vi "Normalize.vi"(8 "error in":errorcluster, 11 "Source graph":cluster{dbl[], dbl[]}[](graph)) -> (0 "error out":errorcluster, 3 "Normalized source graph out":cluster{dbl[], dbl[]}[](graph))   [LabVIEW 2024]
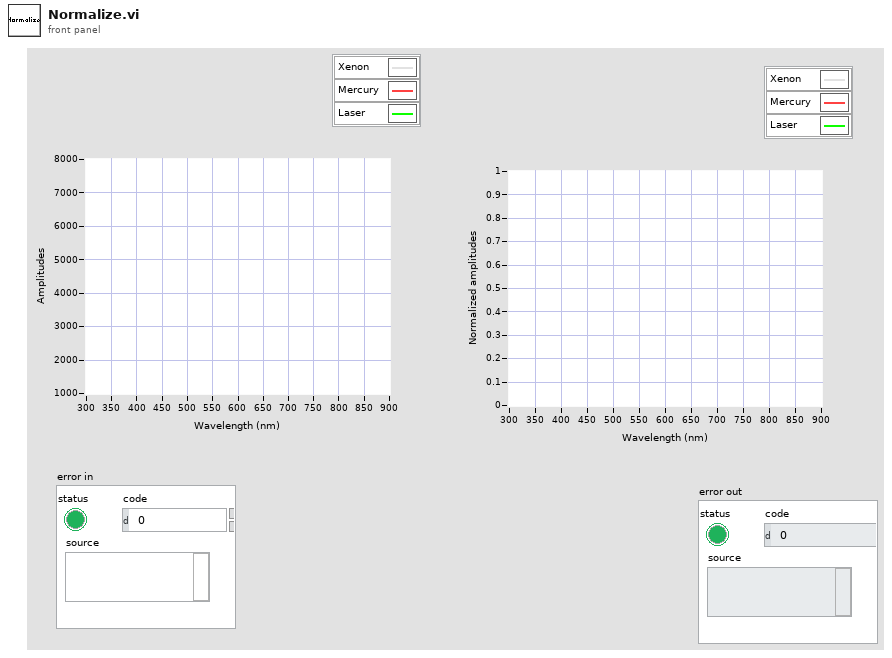
[diagram p1: front panel]
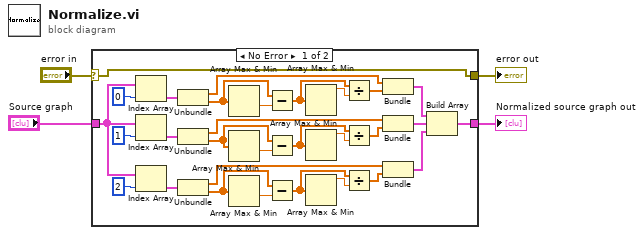
[diagram p0: block diagram]
diagram:
  n1 = case shown="No Error" "error in" {
    selector: "error in" -> [w34 w36]
    tunnel: [w34 w36] -> w3
    tunnel: [w21 w35] -> w2
    tunnel: "Source graph" -> [w30 w35]
    frame No Error {
      n2 = Index Array(array=w30, index=0) -> (element=w29:cluster{dbl[], dbl[]})
      n3 = Index Array(array=w30, index=1) -> (element=w8:cluster{dbl[], dbl[]})
      n4 = Index Array(array=w30, index=2) -> (element=w7:cluster{dbl[], dbl[]})
      n5 = Unbundle(w29) -> (w22:dbl[], w27:dbl[])
      n6 = Unbundle(w8) -> (w15:dbl[], w20:dbl[])
      n7 = Unbundle(w7) -> (w9:dbl[], w14:dbl[])
      n8 = Array Max & Min(array=w27) -> (min value=w26:dbl)  [unwired: 3 out]
      n9 = Array Max & Min(array=w20) -> (min value=w19:dbl)  [unwired: 3 out]
      n10 = Array Max & Min(array=w14) -> (min value=w13:dbl)  [unwired: 3 out]
      n11 = Subtract(x=w27, y=w26) -> (x-y=w25:dbl[])
      n12 = Subtract(x=w20, y=w19) -> (x-y=w18:dbl[])
      n13 = Subtract(x=w14, y=w13) -> (x-y=w12:dbl[])
      n14 = Array Max & Min(array=w25) -> (max value=w24:dbl)  [unwired: 3 out]
      n15 = Array Max & Min(array=w18) -> (max value=w17:dbl)  [unwired: 3 out]
      n16 = Array Max & Min(array=w12) -> (max value=w11:dbl)  [unwired: 3 out]
      n17 = Divide(x=w25, y=w24) -> (x/y=w23:dbl[])
      n18 = Divide(x=w18, y=w17) -> (x/y=w16:dbl[])
      n19 = Divide(x=w12, y=w11) -> (x/y=w10:dbl[])
      n20 = Bundle(w22, w23) -> (w28:cluster{dbl[], dbl[]})  [unwired: 1 in]
      n21 = Bundle(w15, w16) -> (w6:cluster{dbl[], dbl[]})  [unwired: 1 in]
      n22 = Bundle(w9, w10) -> (w5:cluster{dbl[], dbl[]})  [unwired: 1 in]
      n23 = Build Array(w28, w6, w5) -> (w21:cluster{dbl[], dbl[]}[])
    }
    frame Error {
    }
  }
  "Normalized source graph out" <- w2
  "error out" <- w3
